vi "Start Acquisition.vi"(8 "error in":errorcluster, 10 "DAQmx Analog Channels":tag[](array[tag])) -> (0 "error out":errorcluster)   [LabVIEW 2020, in "UI.lvlib"]
doc: "使用するDAQ物理チャンネルを送ってデータ集録を開始します。\n\n_____\nCreated using DQMH Framework: Event Scripter 7.1.2.1547."
uses:
  UI.lvlib
  Start Acquisition Argument--cluster.ctl
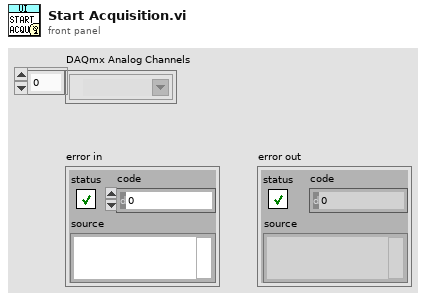
[diagram p1: front panel]
types:
  T1 = typedef "UI.lvlib/Start Acquisition Argument--cluster.ctl" = cluster{"DAQmx Analog Channels":tag[]}
  T2 = typedef "UI.lvlib/Broadcast Events--cluster.ctl" = cluster{"Module Did Init":refnum<user-event>, "Status Updated":refnum<user-event>, "Error Reported":refnum<user-event>, "Module Did Stop":refnum<user-event>, "Update Module Execution Status":refnum<user-event>, "Start Acquisition":refnum<user-event>}
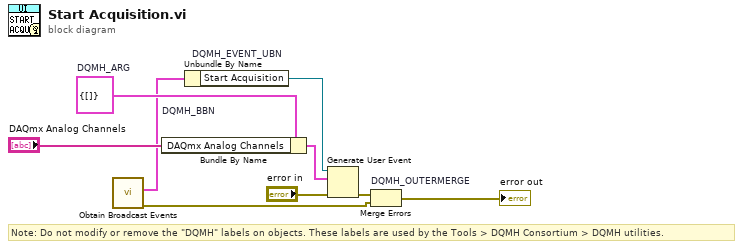
[diagram p0: block diagram]
diagram:
  w4 = T1 {"DAQmx Analog Channels"=[]}  # DQMH_ARG
  # "Note: Do not modify or remove the \"DQMH\" labels on objects. These labels are used by the Tools > DQMH Consortium > DQMH utilities."
  n1 = call "Obtain Broadcast Events.vi"() -> ("error out"=w2:errorcluster, "UI Broadcast Events"=w1:T2)  [unwired: 10 in]
  n2 = Bundle By Name "DQMH_BBN"(cluster=w4, "DAQmx Analog Channels"="DAQmx Analog Channels") -> (w7:T1)
  n3 = Unbundle By Name "DQMH_EVENT_UBN"(w1) -> ("Start Acquisition"=w6:refnum<user-event>)
  n4 = Generate User Event(user event=w6, event data cluster=w7, error in="error in") -> (error out=w5:errorcluster)  [unwired: 1 in, 1 out]
  n5 = Merge Errors "DQMH_OUTERMERGE"(w5, w2) -> (→"error out":errorcluster)
